vi "Standard Deviation .vi"() -> ()   [LabVIEW 2016]
uses:
  <vilib>/Utility/file.llb/Read From Spreadsheet File (DBL).vi
  <vilib>/Analysis/NI_AALBase.lvlib
panel:
  in  "file path":path
  out "Standard Deviation":cluster{"X":dbl, "Y":dbl}={"X"=0.0018340219092498708, "Y"=0.0008201995322957324}
  out "Std":dbl[](array[numeric])=[0.0018340219092498708, 0.0008201995322957324]
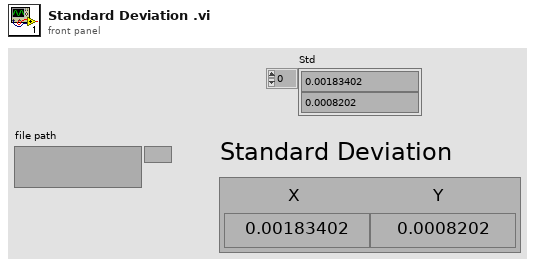
[diagram p1: front panel]
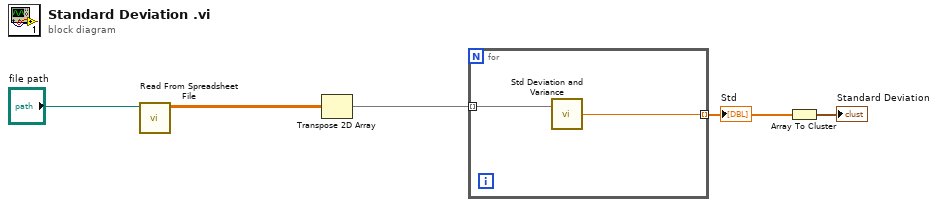
[diagram p0: block diagram]
diagram:
  n1 = call-poly <vilib>:"Read From Spreadsheet File.vi"("file path (dialog if empty)"="file path") -> ("all rows"=w4:dbl[][])  [unwired: 6 in, 4 out]
  n2 = Transpose 2D Array(2D array=w4) -> (transposed array=w5:dbl[][])
  n3 = for {
    tunnel: [w7] -> w3 mode=indexing
    tunnel: w5 -> [w6] mode=indexing
    n4 = call <vilib>:"Std Deviation and Variance.vi"("X"=w6) -> ("standard deviation"=w7:dbl)  [unwired: 1 in, 2 out]
  }
  "Std" <- w3
  n5 = Array To Cluster(array=w3) -> (cluster=→"Standard Deviation":cluster{"[0]":dbl, "[1]":dbl})
